vi "InjectObjectReference.vi"(6 "Dynamic Dispatch":bool, 8 "error in (no error)":errorcluster, 11 "CreateInterface in":refnum<class "CreateInterface.lvclass">) -> (0 "error out":errorcluster, 3 "CreateInterface out":refnum<class "CreateInterface.lvclass">)   [LabVIEW 2020, in "Mermaid.lvlib" / "CreateInterface.lvclass"]
uses:
  CreateInterface.lvclass
  CreateInterface.lvclass/CreateInterface.ctl
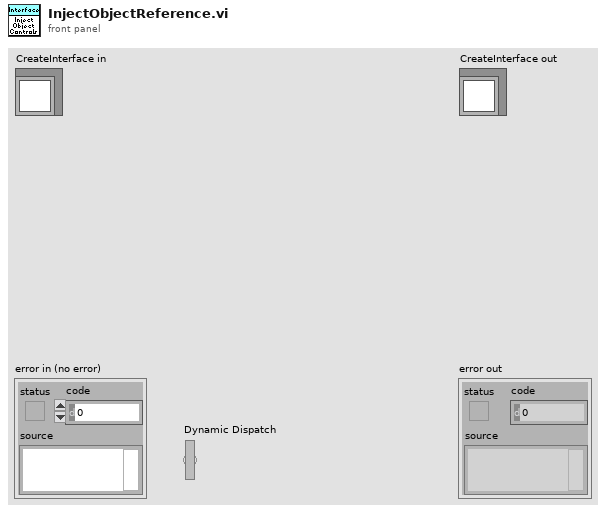
[diagram p1: front panel]
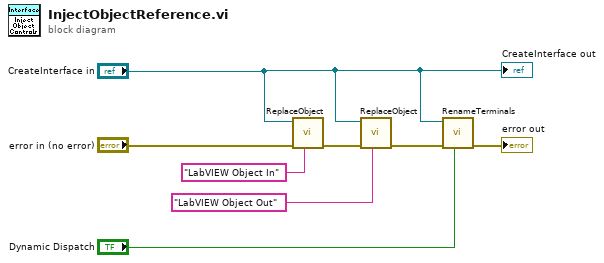
[diagram p0: block diagram]
diagram:
  n1 = call "ReplaceObject.vi"("name/order"="LabVIEW Object In", "error in (no error)"="error in (no error)", "CreateInterface in"="CreateInterface in") -> ("error out"=w6:errorcluster)  [unwired: 8 in]
  n2 = call "ReplaceObject.vi"("name/order"="LabVIEW Object Out", "error in (no error)"=w6, "CreateInterface in"="CreateInterface in") -> ("error out"=w4:errorcluster)  [unwired: 8 in]
  n3 = call "RenameTerminals.vi"("Dynamic Dispatch"="Dynamic Dispatch", "error in (no error)"=w4, "CreateInterface in"="CreateInterface in") -> ("error out"=→"error out":errorcluster)  [unwired: 8 in]
  "CreateInterface out" <- "CreateInterface in"
